vi "AVS_GetScopeData.vi"(0 "a_hDevice":i32, 7 "a_pTimeLabel":u32, 11 "a_pSpectrum":dbl[](array[numeric])) -> (4 "Output Value":i32, 8 "a_pTimeLabel":u32, 15 "a_pSpectrum":dbl[](array[numeric]))   [LabVIEW 2014, in "AvaSpec.lvlib" / "Avantes Spectrometer Functions.lvlib"]
uses:
  Avantes Spectrometer Functions.lvlib
  AS5216.dll
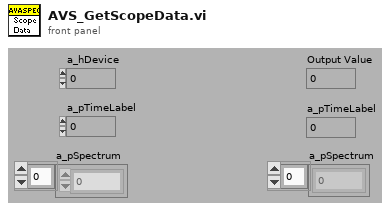
[diagram p1: front panel]
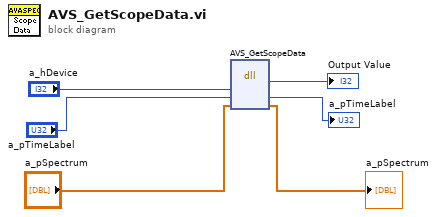
[diagram p0: block diagram]
diagram:
  n1 = dll-call lib="C:/Users/Daniel/Dropbox/CLTC/avantesSpectrometer/Libraries/AS-5216-DLL/polling_mc/AS5216.dll" fn="AVS_GetScopeData"("a_hDevice"="a_hDevice", "a_pTimeLabel"="a_pTimeLabel", "a_pSpectrum"="a_pSpectrum") -> (→"Output Value":i32, "a_pTimeLabel"=→"a_pTimeLabel":u32, "a_pSpectrum"=→"a_pSpectrum":dbl[])  [unwired: 4 in, 2 out]
